vi "Visualize.vi"   [LabVIEW 2014]
uses:
  Visualization.lvlib
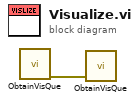
[diagram p0: block diagram]
diagram:
  n1 = call "ObtainVisQue.vi"() -> ("error out"=w1:errorcluster)  [unwired: 10 in, 1 out]
  n2 = call "ObtainVisQue.vi"("error in (no error)"=w1) -> ()  [unwired: 9 in, 2 out]
